vi "Reset.vi"(8 "error in (no error)":errorcluster, 11 "MC switch refnum in":refnum<k24>) -> (0 "error out":errorcluster, 3 "MC switch refnum out":refnum<k24>)   [LabVIEW 2019, in "Minicircuit RF Switch Box.lvlib"]
doc: "Resets the instrument and then sends a set of default setup commands to the instrument."
uses:
  <instrlib>/LV_Minicircuit_RF_Switch/Minicircuit RF Switch Box.lvlib
  C:/Program Files (x86)/National Instruments/LabVIEW 2019/instr.lib/LV_Minicircuit_RF_Switch/mcl_RF_Switch_Controller_NET45.dll
  mcl_RF_Switch_Controller_NET45.dll
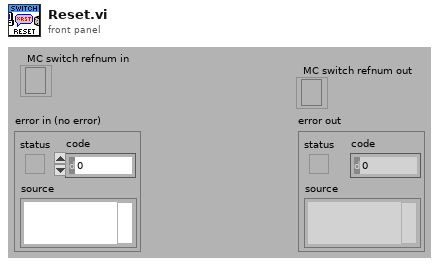
[diagram p1: front panel]
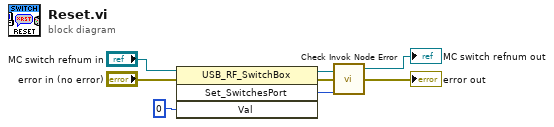
[diagram p0: block diagram]
diagram:
  n1 = invoke class="USB_RF_SwitchBox" method="Set_SwitchesPort"(reference="MC switch refnum in", error in="error in (no error)", "Val"=u8 0) -> (reference out=w6:refnum<k24>, error out=w5:errorcluster, "Set_SwitchesPort"=w4:i32)  [unwired: 1 in, 1 out]
  n2 = call <instrlib>:"Check Invok Node Error.vi"("Connect"=w4, "error in (no error)"=w5, "MC switch refnum in"=w6) -> ("error out"=→"error out":errorcluster, "MC switch refnum out"=→"MC switch refnum out":refnum<k24>)  [unwired: 1 in]
